vi "Save_meas_data.vi"(0 "Path":path, 5 "Meas. Param. Data Cluster":T2, 7 "Data":T1, 9 "k":dbl, 11 "error in":errorcluster) -> (15 "error out":errorcluster)   [LabVIEW 2021]
uses:
  Data.ctl
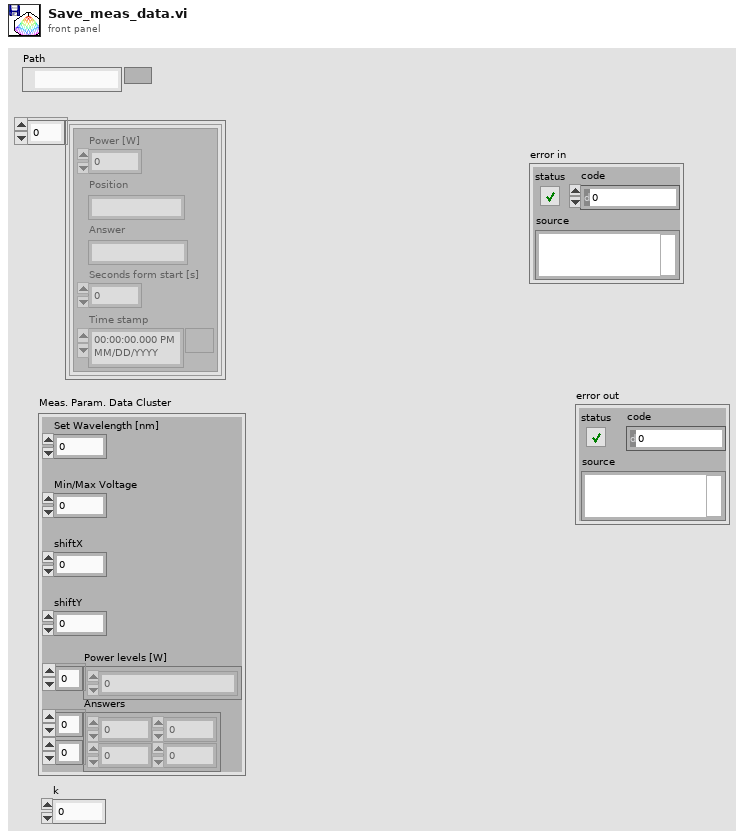
[diagram p1: front panel]
types:
  T1 = typedef "Data.ctl" = cluster{cluster{"Power [W]":dbl, "Position":string, "Answer":string, "Seconds form start [s]":dbl, "Time stamp":timestamp}}[]
  T2 = cluster{"Set Wavelength [nm]":dbl, "Min/Max Voltage":dbl, "shiftX":dbl, "shiftY":dbl, "Power levels [W]":dbl[], "Answers":i32[][]}
  T3 = enum16{"open", "replace", "create", "open or create", "replace or create", "replace or create with confirmation"}
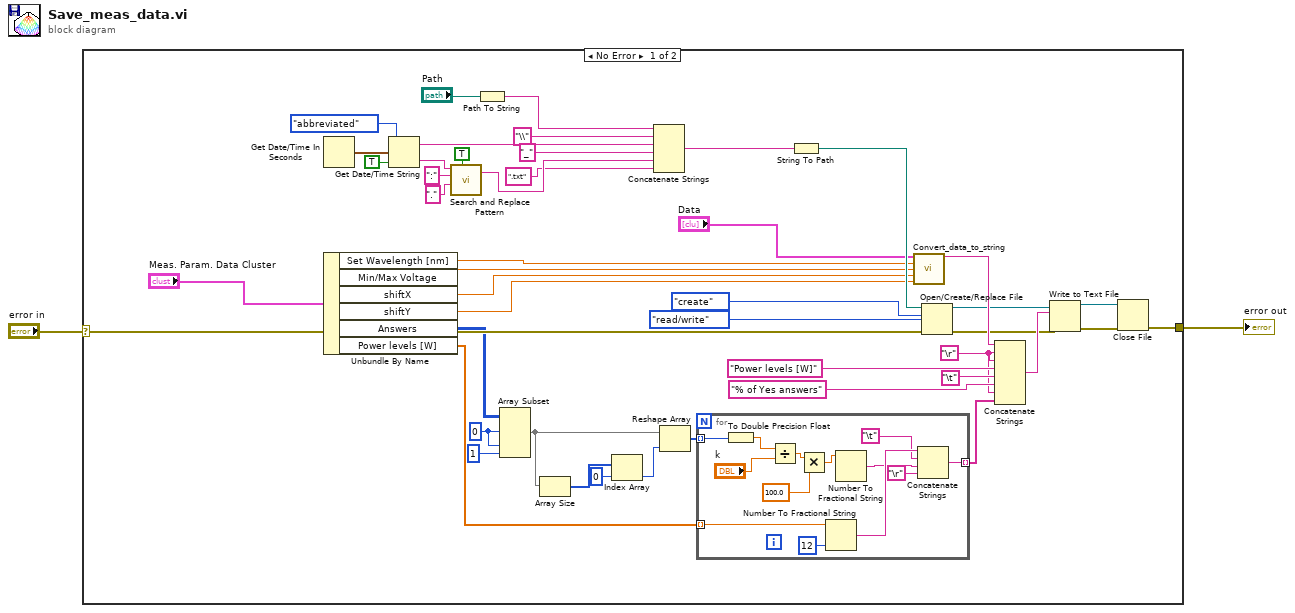
[diagram p0: block diagram]
diagram:
  n1 = case shown="No Error" "error in" {
    selector: "error in" -> [w23 w62]
    tunnel: [w46 w62] -> w2
    frame No Error {
      w10 = "\r"
      w14 = 0 ("index")
      n2 = Get Date/Time In Seconds() -> (seconds since 1Jan1904=w25:timestamp)
      n3 = Unbundle By Name("Meas. Param. Data Cluster") -> ("Set Wavelength [nm]"=w21:dbl, "Min/Max Voltage"=w18:dbl, "shiftX"=w19:dbl, "shiftY"=w20:dbl, "Answers"=w15:i32[][], "Power levels [W]"=w9:dbl[])
      n4 = Get Date/Time String(date format (0)=enum16{"short", "long", "abbreviated"}."abbreviated", seconds (now)=w25, want seconds? (F)=TRUE) -> (date string=w28:string, time string=w44:string)
      n5 = call <vilib>:"Search and Replace Pattern.vi"("string"=w44, "regular expression (\"\")"=":" ("regular expression (\"\")"), "replace string (\"\")"="." ("replace string (\"\")"), "replace all? (F)"=TRUE) -> ("result string"=w43:string)  [unwired: 1 in, 1 out]
      n6 = Path To String(path="Path") -> (string=w36:string)
      n7 = Array Subset(array=w15, index (row)=w14, index (col)=w14, length (col)=1 ("length")) -> (w6:i32[][])  [unwired: 1 in]
      n8 = Array Size(array=w6) -> (size(s)=w5:i32[])
      n9 = Index Array(array=w5, index=0) -> (element=w4:i32)
      n10 = Concatenate Strings(w36, "\\" ("string"), w28, "_", w43, ".txt" ("string")) -> (w34:string)
      n11 = Reshape Array(w6, w4) -> (w7:i32[])
      n12 = for {
        tunnel: w9 -> [w60] mode=indexing
        tunnel: [w61] -> w8 mode=indexing
        tunnel: w7 -> [w52] mode=indexing
        n13 = To Double Precision Float(number=w52) -> (double precision float=w51:dbl)
        n14 = Divide(x=w51, y="k") -> (x/y=w54:dbl)
        n15 = Multiply(x=w54, y=100.0) -> (x*y=w55:dbl)
        n16 = Number To Fractional String(number=w60, precision (6)=i16 12) -> (F-format string=w59:string)  [unwired: 2 in]
        n17 = Number To Fractional String(number=w55) -> (F-format string=w56:string)  [unwired: 3 in]
        n18 = Concatenate Strings(w59, "\t", w56, "\r") -> (w61:string)
      }
      n19 = String To Path(string=w34) -> (path=w38:path)
      n20 = call "Convert_data_to_string.vi"("Data"="Data", "Wavelenght [nm]"=w21, "Min/Max Voltage [V]"=w18, "X Shift [V]"=w19, "Y Shift [V]"=w20) -> ("spreadsheet string"=w48:string)  [unwired: 10 in]
      n21 = Open/Create/Replace File(file path (use dialog)=w38, error in=w23, operation (0:open)=T3."create", access (0:read/write)=enum16{"read/write", "read-only", "write-only"}."read/write") -> (refnum out=w30:refnum<file>, error out=w39:errorcluster)  [unwired: 2 in, 1 out]
      n22 = Concatenate Strings(w48, w10, w10, "Power levels [W]" ("string"), "\t", "% of Yes answers" ("string"), w10, w8) -> (w47:string)
      n23 = Write to Text File(file (use dialog)=w30, text=w47, error in=w39) -> (refnum out=w24:refnum<file>, error out=w40:errorcluster)  [unwired: 1 in, 1 out]
      n24 = Close File(refnum=w24, error in=w40) -> (error out=w46:errorcluster)  [unwired: 1 out]
    }
    frame Error {
    }
  }
  "error out" <- w2
